vi "ZAlign_SetOrigin0.vi"(8 "error in (no error)":errorcluster, 11 "Panel in":refnum<vi>) -> (0 "error out":errorcluster, 3 "reference out":refnum<vi>)   [LabVIEW 2014, in "ZAlign.lvlib"]
doc: "ZAlign.lvlib:ZAlign_SetOrigin0.vi\n----------------------------------------------\nSet Origin to 0\n\nInputs:\n---------------------\n- error in (no error) : Cluster; \n- Panel in : Refnum; \n\nOutputs:\n---------------------\n- error out : Cluster; \n- reference out : Refnum; \n\n----------------------------------------------\n16/03/2015\nZühlke Engineering AG\nCH-8952 Schlieren\nwww.zuehlke.com"
uses:
  ZAlign.lvlib
  <vilib>/Utility/miscctls.llb/LVPointTypeDef.ctl
panel:
  # "Connector Pane"
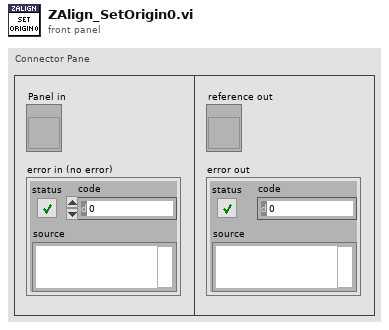
[diagram p1: front panel]
types:
  T1 = typedef "LVPointTypeDef.ctl" = cluster{"Horizontal":i16, "Vertical":i16}
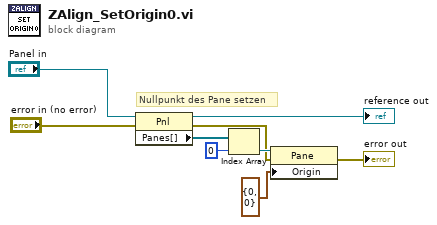
[diagram p0: block diagram]
diagram:
  # "Nullpunkt des Pane setzen"
  n1 = property class="Pnl"(reference="Panel in", error in="error in (no error)") -> (reference out=→"reference out":refnum<vi>, error out=w1:errorcluster, "Panes[]"=w2:refnum<vi>[])
  n2 = Index Array(array=w2, index=0) -> (element=w4:refnum<vi>)
  n3 = property class="Pane"(reference=w4, error in=w1, "Origin"=T1 {"Horizontal"=0, "Vertical"=0}) -> (error out=→"error out":errorcluster)  [unwired: 1 out]
